vi "WPI_Camera CGI Parse for WB.vi"(11 "String":string="fixed_indoor") -> (1 "Numeric":i32, 2 "enum":T1)   [LabVIEW 2017]
uses:
  <vilib>/Rock Robotics/WPI/Camera/WPI_CameraWhite Balance Values.ctl
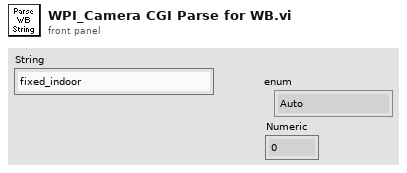
[diagram p1: front panel]
types:
  T1 = typedef "WPI_CameraWhite Balance Values.ctl" = enum16{"Auto", "Fixed indoor", "Fixed outdoor 1", "Fixed outdoor 2", "Fixed fluorescent 1", "Fixed fluorescent 2", "Hold current", "Custom"}
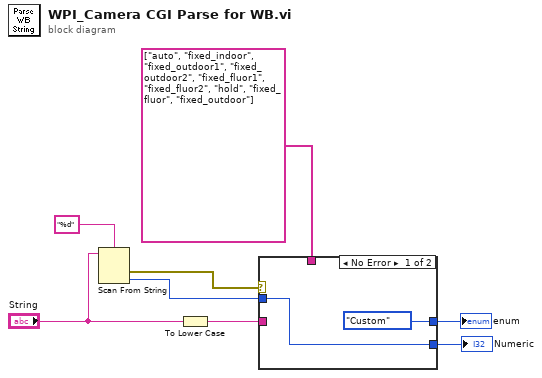
[diagram p0: block diagram]
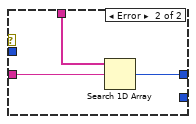
[diagram p2: hidden frame]
diagram:
  n1 = Scan From String(format string="%d", input string="String") -> (error out=w4:errorcluster, output 1=w2:i32)  [unwired: 3 in, 2 out]
  n2 = To Lower Case(string="String") -> (all lower case string=w7:string)
  n3 = case shown="No Error" w4 {
    tunnel: string[] ["auto", "fixed_indoor", "fixed_outdoor1", "fixed_outdoor2", "fixed_fluor1", "fixed_fluor2", "hold", "fixed_fluor", "fixed_outdoor"] ("Array") -> [_ w13]
    tunnel: w7 -> [_ w12]
    tunnel: [WPI_CameraWhite_Balance_Values."Custom" ("enum") w11] -> w3
    tunnel: w2 -> [w10 _]
    tunnel: [w10 _] -> w1
    frame No Error {
    }
    frame Error {
      n4 = Search 1D Array(1D array=w13, element=w12) -> (index of element=w11:i32)  [unwired: 1 in]
    }
  }
  "enum" <- w3
  "Numeric" <- w1
